vi "Click Event.vi"(8 "error in (no error)":errorcluster, 9 "Event Data":variant, 11 "object in":refnum<class "Vi_Button.lvclass">) -> (0 "error out":errorcluster, 2 "Value Changed ?":bool, 3 "object out":refnum<class "Vi_Button.lvclass">)   [LabVIEW 2012, in "Vi_Button.lvclass"]
uses:
  Vi_Button.lvclass
  Vi_Button.lvclass/Vi_Button.ctl
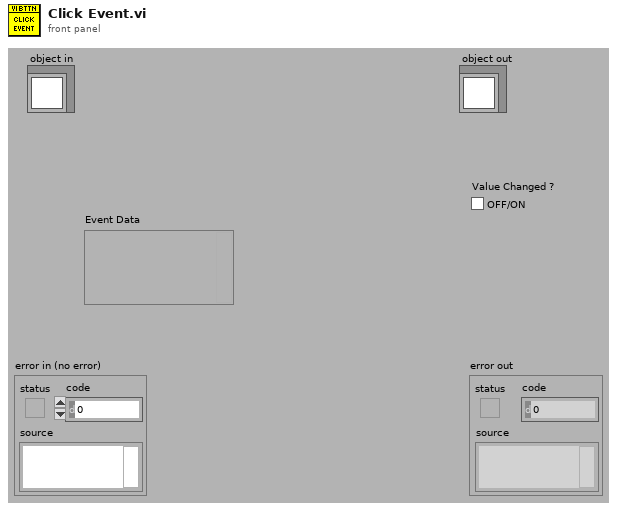
[diagram p1: front panel]
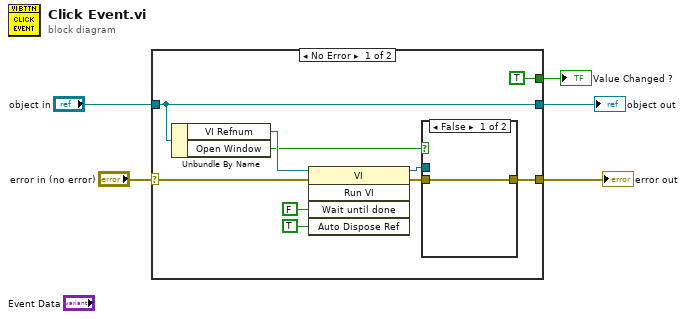
[diagram p0: block diagram]
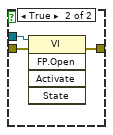
[diagram p2: hidden frame]
diagram:
  n1 = case shown="No Error" "error in (no error)" {
    selector: "error in (no error)" -> [w8 w21]
    tunnel: [w7 w21] -> w4
    tunnel: [w9 w20] -> w2
    tunnel: "object in" -> [w9 w20]
    tunnel: [TRUE _] -> w1
    frame No Error {
      n2 = Unbundle By Name(w9) -> ("VI Refnum"=w15:refnum<vi>, "Open Window"=w10:bool)
      n3 = invoke class="VI" method="Run VI"(reference=w15, error in=w8, "Wait until done"=FALSE ("Wait Until Done"), "Auto Dispose Ref"=TRUE ("Auto Dispose Reference")) -> (reference out=w12:refnum<vi>, error out=w11:errorcluster)  [unwired: 1 in, 3 out]
      n4 = case shown="False" w10 {
        tunnel: w12 -> [_ w19]
        tunnel: w11 -> [w16 w18]
        tunnel: [w16 w17] -> w7
        frame False {
        }
        frame True {
          n5 = invoke class="VI" method="FP.Open"(reference=w19, error in=w18) -> (error out=w17:errorcluster)  [unwired: 3 in, 4 out]
        }
      }
    }
    frame Error {
    }
  }
  "error out" <- w4
  "object out" <- w2
  "Value Changed ?" <- w1
